vi "Init.vi"(9 "Dt":dbl, 10 "Size":i32, 11 "LRS in":refnum<class "LRS.lvclass">) -> (3 "LRS out":refnum<class "LRS.lvclass">)   [LabVIEW 2013, in "Exponential Fit Library.lvlib" / "LRS.lvclass"]
doc: "From Everest and Atkinson [2008]: the sums over t and t^2 can be determined apriori and therefore we only need to do them when we initialize."
uses:
  LRS.lvclass
  Fit Exponential.lvclass
  LRS.lvclass/LRS.ctl
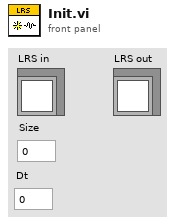
[diagram p1: front panel]
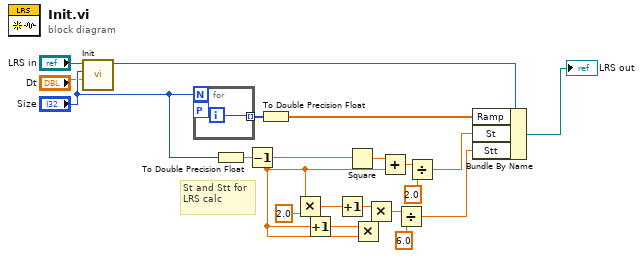
[diagram p0: block diagram]
diagram:
  # "St and Stt for LRS calc"
  n1 = call-parent "Init.vi"("Dt"="Dt", "Size"="Size", "Fit Exponential in"="LRS in") -> ("Fit Exponential out"=w6:refnum<class "LRS.lvclass">)  [unwired: 8 in]
  n2 = for {
    N: "Size" -> [_]
    tunnel: [w22] -> w20 mode=indexing
    workers-P: _ -> [_]
    i -> [w22]
  }
  n3 = To Double Precision Float(number="Size") -> (double precision float=w19:dbl)
  n4 = Decrement(x=w19) -> (x-1=w18:dbl)
  n5 = To Double Precision Float(number=w20) -> (double precision float=w5:dbl[])
  n6 = Multiply(x=w18, y=2.0) -> (x*y=w12:dbl)
  n7 = Increment(x=w18) -> (x+1=w13:dbl)
  n8 = Increment(x=w12) -> (x+1=w15:dbl)
  n9 = Square(x=w18) -> (x^2=w8:dbl)
  n10 = Multiply(x=w13, y=w18) -> (x*y=w14:dbl)
  n11 = Multiply(x=w15, y=w14) -> (x*y=w16:dbl)
  n12 = Add(x=w8, y=w18) -> (x+y=w9:dbl)
  n13 = Divide(x=w16, y=6.0) -> (x/y=w3:dbl)
  n14 = Divide(x=w9, y=2.0) -> (x/y=w4:dbl)
  n15 = Bundle By Name(cluster=w6, "Ramp"=w5, "St"=w4, "Stt"=w3) -> (→"LRS out":refnum<class "LRS.lvclass">)
